vi "Build_2019_Version.vi"() -> ()   [LabVIEW 2020]
panel:
  out "error out":errorcluster
  out "Array":T1(array[cluster])
  out "Warnings":string
  # "Open ME35 to make sure things are loaded in memory"
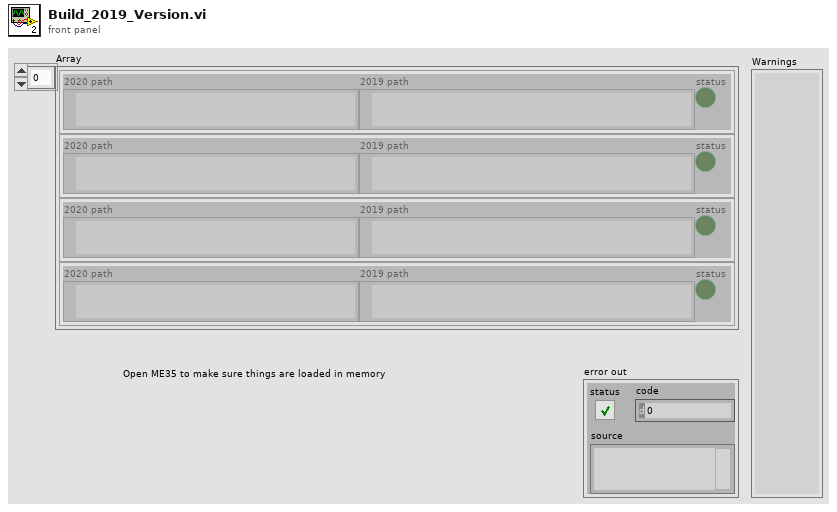
[diagram p1: front panel]
types:
  T1 = cluster{"2020 path":path, "2019 path":path, "status":bool}[]
  T2 = enum8{"Only include commented out diagrams if diagram already loaded", "Never include commented out diagrams", "Always include commented out diagrams"}
  T3 = cluster{path, "appended path":path, "status":bool}
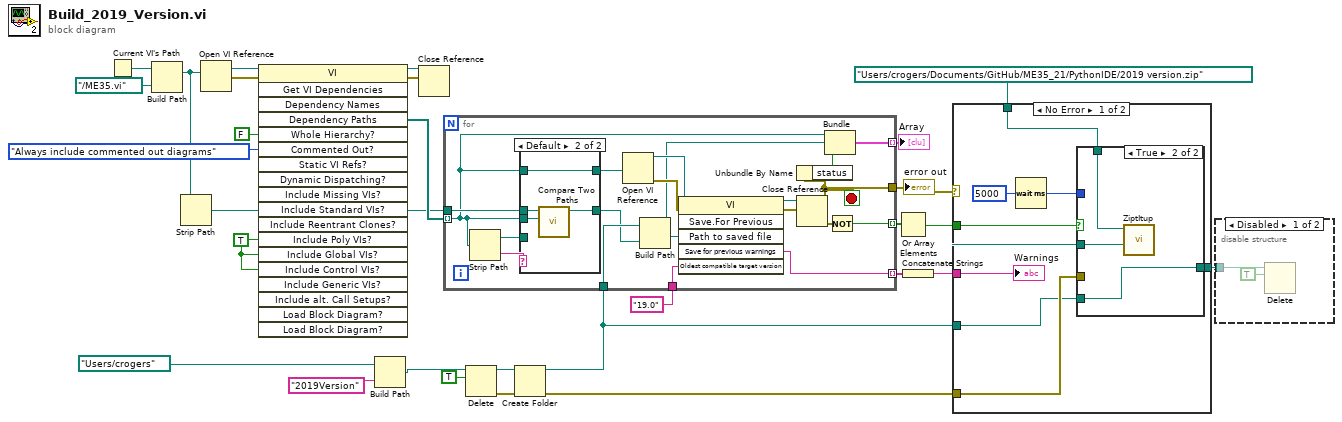
[diagram p0: block diagram]
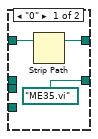
[diagram p5: hidden frame]
diagram:
  w11 = TRUE ("Whole Hierarchy?")
  n1 = Current VI's Path() -> (path=w28:path)
  n2 = Build Path(base path=w28, name or relative path=path "../ME35.vi") -> (appended path=w5:path)
  n3 = Strip Path(path=w5) -> (stripped path=w4:path)  [unwired: 1 out]
  n4 = Open VI Reference(vi path=w5) -> (vi reference=w26:refnum<vi>, error out=w10:errorcluster)  [unwired: 5 in]
  n5 = invoke class="VI" method="Get VI Dependencies"(reference=w26, error in=w10, "Whole Hierarchy?"=FALSE, "Commented Out?"=T2."Always include commented out diagrams" ("Commented Out Diagrams?"), "Include Poly VIs?"=w11, "Include Global VIs?"=w11, "Include Control VIs?"=w11) -> (reference out=w12:refnum<vi>, error out=w9:errorcluster, "Dependency Paths"=w24:path[])  [unwired: 12 in, 16 out]
  n6 = Build Path(base path=path "/Users/crogers" ("name or relative path"), name or relative path="2019Version" ("Target Version")) -> (appended path=w17:path)
  n7 = Close Reference(reference=w12, error in (no error)=w9) -> ()  [unwired: 1 out]
  n8 = Delete(path (use dialog)=w17, entire hierarchy (F)=TRUE) -> (deleted path=w6:path, error out=w16:errorcluster)  [unwired: 3 in, 1 out]
  n9 = Create Folder(path (use dialog)=w6) -> (created path=w3:path)  [unwired: 2 in, 2 out]
  n10 = for {
    tunnel: w4 -> [w46]
    tunnel: w24 -> [w31] mode=indexing
    tunnel: w3 -> [w43]
    tunnel: "19.0" ("Target Version") -> [w45]
    tunnel: [w44] -> w22 mode=indexing
    tunnel: [w34] -> w20 mode=indexing
    tunnel: [w35] -> w15 mode=indexing
    tunnel: [w29] -> w1
    stop <- w29 stop-if-true
    n11 = Strip Path(path=w31) -> (stripped path=w32:path, name=w33:string)
    n12 = case shown="Default" w33 {
      tunnel: w46 -> [_ w53]
      tunnel: [path "ME35.vi" ("name or relative path") w52] -> w42
      tunnel: w31 -> [_ w51]
      tunnel: w32 -> [_ _]
      tunnel: w31 -> [w48 w50]
      tunnel: [w47 w50] -> w30
      frame "0" {
        n13 = Strip Path(path=w48) -> (stripped path=w47:path)  [unwired: 1 out]
      }
      frame Default {
        n14 = call <vilib>:"Compare Two Paths.vi"("Path 2"=w51, "Path 1"=w53) -> ("Relative Path from 1 to 2"=w52:path)  [unwired: 6 in, 3 out]
      }
    }
    n15 = Open VI Reference(vi path=w30) -> (vi reference=w41:refnum<vi>, error out=w38:errorcluster)  [unwired: 5 in]
    n16 = Build Path(base path=w43, name or relative path=w42) -> (appended path=w37:path)
    n17 = invoke class="VI" method="Save.For Previous"(reference=w41, error in=w38, "Path to saved file"=w37, "Oldest compatible target version"=w45) -> (reference out=w40:refnum<vi>, error out=w39:errorcluster, "Save for previous warnings"=w44:string)  [unwired: 2 in, 3 out]
    n18 = Close Reference(reference=w40, error in (no error)=w39) -> (error out=w29:errorcluster)
    n19 = Unbundle By Name(w29) -> ("status"=w36:bool)
    n20 = Bundle(w31, "appended path"=w37, "status"=w36) -> (w35:T3)  [unwired: 1 in]
    n21 = Not(x=w29) -> (.not. x?=w34:bool)
  }
  "Array" <- w15
  "error out" <- w1
  n22 = Or Array Elements(Boolean array=w20) -> (logical OR=w14:bool)
  n23 = Concatenate Strings(w22) -> (w13:string)
  n24 = case shown="No Error" w1 {
    tunnel: w16 -> [w61 _]
    tunnel: w14 -> [w60 _]
    tunnel: w13 -> [w59 _]
    tunnel: path "/Users/crogers/Documents/GitHub/ME35_21/PythonIDE/2019 version.zip" ("name or relative path") -> [w58 _]
    tunnel: [w57 w66] -> w7
    tunnel: w3 -> [w56 w66]
    frame No Error {
      n25 = Wait (ms)(milliseconds to wait=u32 5000) -> (millisecond timer value=w54:u32)
      n26 = case shown="True" w60 {
        tunnel: w56 -> [_ w65]
        tunnel: w61 -> [_ _]
        tunnel: w58 -> [_ w64]
        tunnel: [w62 w63] -> w57
        tunnel: w56 -> [w62 w63]
        tunnel: w54 -> [_ _]
        frame False {
        }
        frame True {
          n27 = call "ZiptItup.vi"("Folder to zip"=w65, "Zip file"=w64) -> ()  [unwired: 8 in, 2 out]
        }
      }
      "Warnings" <- w59
    }
    frame Error {
    }
  }
  n28 = disable-structure shown="Disabled" {
    disable-tunnel: w7 -> [w67 _]
    frame Disabled {
      n29 = Delete(path (use dialog)=w67, entire hierarchy (F)=TRUE) -> ()  [unwired: 3 in, 3 out]
    }
    frame Enabled {
    }
  }
